vi "_TangoReadStateScalarAttribute.vi"(3 "error in":errorcluster, 4 "attribute name":string, 5 "device name":string) -> (0 "error out":errorcluster, 1 "setpoint":T1=enum."UNKNOWN", 2 "value":T1=enum."UNKNOWN")   [LabVIEW 2014, in "tango.lvlib"]
uses:
  tango.lvlib
  Common VIs/Typedefs/_TangoState_t.ctl
  Common VIs/Typedefs/_AttributeDataType_t.ctl
  Extractors/base/toStateScalar.vi
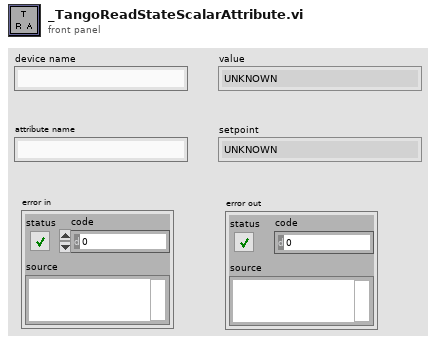
[diagram p1: front panel]
types:
  T1 = typedef "tango.lvlib/_TangoState_t.ctl" = enum32{"ON", "OFF", "CLOSE", "OPEN", "INSERT", "EXTRACT", "MOVING", "STANDBY", "FAULT", "INIT", "RUNNING", "ALARM", "DISABLE", "UNKNOWN"}
  T2 = typedef "tango.lvlib/_AttributeDataType_t.ctl" = enum16{"STATE_SCA", "STATE_SPE", "STATE_IMG", "STRING_SCA", "STRING_SPE", "STRING_IMG", "BOOL_SCA", "BOOL_SPE", "BOOL_IMG", "UCHAR_SCA", "UCHAR_SPE", "UCHAR_IMG", "SHORT_SCA", "SHORT_SPE", "SHORT_IMG", "USHORT_SCA", "USHORT_SPE", "USHORT_IMG", "LONG_SCA", "LONG_SPE", "LONG_IMG", "ULONG_SCA", "ULONG_SPE", "ULONG_IMG", "LONG64_SCA", "LONG64_SPE", "LONG64_IMG", "ULONG64_SCA", "ULONG64_SPE", "ULONG64_IMG", "FLOAT_SCA", "FLOAT_SPE", "FLOAT_IMG", "DOUBLE_SCA", "DOUBLE_SPE", "DOUBLE_IMG", "UNKNOWN_DATA_TYPE"}
  T3 = typedef "tango.lvlib/_AttributeQuality_t.ctl" = enum16{"VALID", "INVALID", "ALARM", "CHANGING", "UNKNOWN_QUALITY"}
  T4 = cluster{"device name":string, "attribute name":string, "quality value":T3, "quality string":string, "timestamp":dbl, "dim. x":i32, "dim. y":i32, "value":u8[], "error code":i32, "error stack":string[], "data type":T2}[]
  T5 = cluster{"device name":string, "attribute name":string, "quality value":T3, "quality string":string, "timestamp":dbl, "dim. x":i32, "dim. y":i32, "value":u8[], "error code":i32, "error stack":string[], "data type":T2}
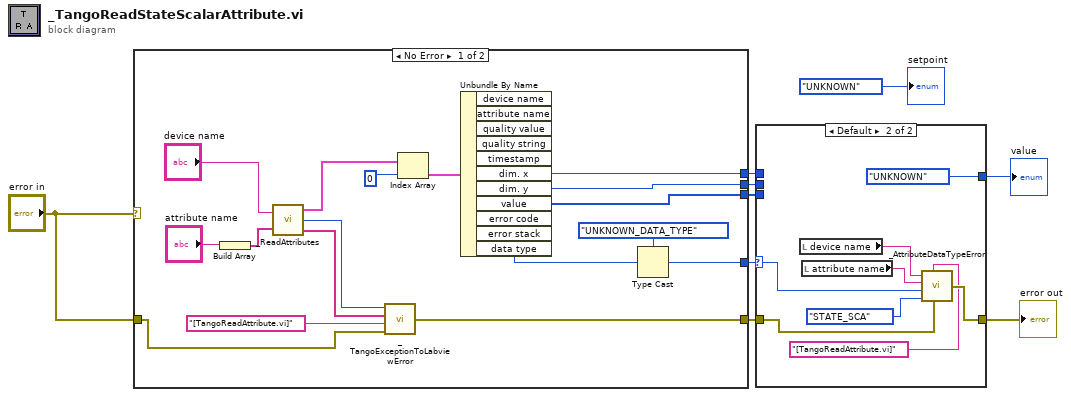
[diagram p0: block diagram]
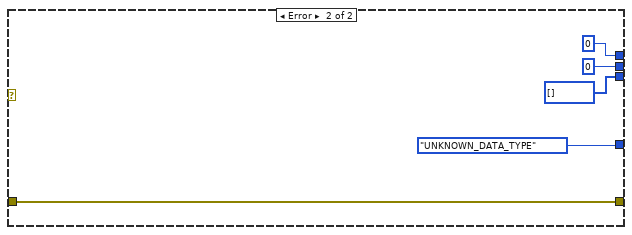
[diagram p2: hidden frame]
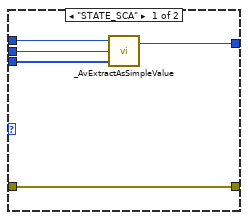
[diagram p3: hidden frame]
diagram:
  n1 = case shown="No Error" "error in" {
    tunnel: [w15 0 ("dim. x")] -> w9
    tunnel: [w14 0 ("dim. y")] -> w8
    tunnel: [w13 u8[] [] ("value")] -> w7
    tunnel: [w12 w31] -> w5
    tunnel: "error in" -> [w11 w31]
    tunnel: [w10 _AttributeDataType_t."UNKNOWN_DATA_TYPE" ("Control")] -> w1
    frame No Error {
      n2 = Build Array("attribute name") -> (w21:string[])
      n3 = call "_ReadAttributes.vi"("device name"="device name", "attribute names"=w21) -> ("attribute values"=w23:T4, "error code"=w16:i32, "error stack"=w17:string[])
      n4 = call "_TangoExceptionToLabviewError.vi"("error in"=w11, "location"="[TangoReadAttribute.vi]", "error stack"=w17, "error code"=w16) -> ("error out"=w12:errorcluster)
      n5 = Index Array(array=w23, index=0 ("indice")) -> (element=w24:T5)
      n6 = Unbundle By Name(w24) -> ("dim. x"=w15:i32, "dim. y"=w14:i32, "value"=w13:u8[], "data type"=w19:T2)  [unwired: 7 out]
      n7 = Type Cast(type=_AttributeDataType_t."UNKNOWN_DATA_TYPE" ("Control"), x=w19) -> (*(type *) &x=w10:T2)
    }
    frame Error {
    }
  }
  n8 = case shown="Default" w1 {
    selector: w1 -> [_ w43]
    tunnel: w9 -> [w36 _]
    tunnel: w8 -> [w35 _]
    tunnel: w7 -> [w34 _]
    tunnel: [w33 _TangoState_t."UNKNOWN" ("Tango Device State")] -> w3
    tunnel: w5 -> [w32 w40]
    tunnel: [w32 w39] -> w4
    frame "STATE_SCA" {
      n9 = call-poly "_AvExtractAsSimpleValue.vi"("value_in"=w34, "dim_y"=w35, "dim_x"=w36) -> ("value_out"=w33:T1)  [unwired: 1 out]
    }
    frame Default {
      n10 = local read "device name"() -> (w41:string)
      n11 = local read "attribute name"() -> (w42:string)
      n12 = call "_AttributeDataTypeError.vi"("error in"=w40, "location"="[TangoReadAttribute.vi]", "user Data Type"=_AttributeDataType_t."STATE_SCA" ("Control"), "actual Data Type"=w43, "attribute name"=w42, "device name"=w41) -> ("error out"=w39:errorcluster)
    }
  }
  "error out" <- w4
  "value" <- w3
  "setpoint" <- _TangoState_t."UNKNOWN" ("Tango Device State")
